vi "Authorization Decode String.vi"(8 "error in (no error)":errorcluster, 10 "RootPathName (C:\\)":string="C:\\", 11 "Encoded String":string) -> (0 "error out":errorcluster, 2 "Property Name":string, 3 "Decoded String":string, 4 "Valid?":bool, 5 "Volume Serial Number (String)":string, 7 "Volume Serial Number (PC)":string)   [LabVIEW 2011]
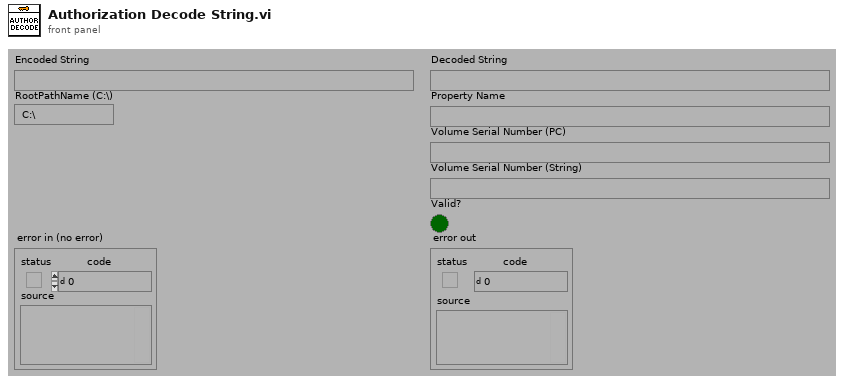
[diagram p1: front panel]
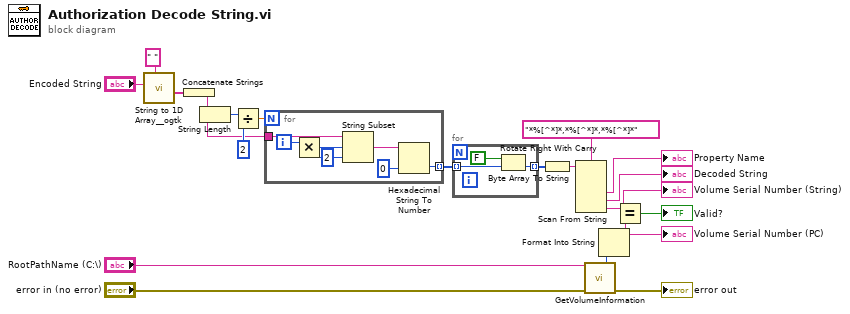
[diagram p0: block diagram]
diagram:
  n1 = call "String to 1D Array__ogtk.vi"("delimiter (Tab)"=" ", "string"="Encoded String") -> ("Array of Strings"=w15:string[])  [unwired: 9 in]
  n2 = Concatenate Strings(w15) -> (w11:string)
  n3 = String Length(string=w11) -> (length=w14:i32)
  n4 = Divide(x=w14, y=2) -> (x/y=w12:dbl)
  n5 = for {
    N: w12 -> [_]
    tunnel: w11 -> [w25]
    tunnel: [w21] -> w10 mode=indexing
    i -> [w22]
    w23 = 2 ("length (rest)")
    n6 = Multiply(x=w22, y=w23) -> (x*y=w24:i32)
    n7 = String Subset(string=w25, offset (0)=w24, length (rest)=w23) -> (substring=w27:string)
    n8 = Hexadecimal String To Number(string=w27, default (0uL)=u8 0 ("default (0 U32)")) -> (number=w21:u8)  [unwired: 1 in, 1 out]
  }
  n9 = for {
    tunnel: w10 -> [w30] mode=indexing
    tunnel: [w29] -> w20 mode=indexing
    n10 = Rotate Right With Carry(2:w30, 3:FALSE ("carry")) -> (0:w29:u8)  [unwired: 1 out]
  }
  n11 = Byte Array To String(unsigned byte array=w20) -> (string=w19:string)
  n12 = Scan From String(format string="*%[^*]*,*%[^*]*,*%[^*]*", input string=w19) -> (output 1=→"Property Name":string, output 2=→"Decoded String":string, output 3=w3:string)  [unwired: 5 in, 3 out]
  "Volume Serial Number (String)" <- w3
  n13 = call "GetVolumeInformation.vi"("RootPathName (C:\\)"="RootPathName (C:\\)", "error in (no error)"="error in (no error)") -> ("VolumeSerialNumber"=w7:u32, "error out"=→"error out":errorcluster)  [unwired: 7 in, 5 out]
  n14 = Format Into String(w7) -> (resulting string=w2:string)  [unwired: 3 in, 1 out]
  "Volume Serial Number (PC)" <- w2
  n15 = Equal?(x=w3, y=w2) -> (x = y?=→"Valid?":bool)
